vi "Test Data Trimming.vi"() -> ()   [LabVIEW 2018]
panel:
  out "time":dbl
  out "array for saving":sgl[](array[numeric])
  in  "start pixel":i32
  in  "#A-lines per B-line":i32=2048
  in  "#pixels to save":i32=200
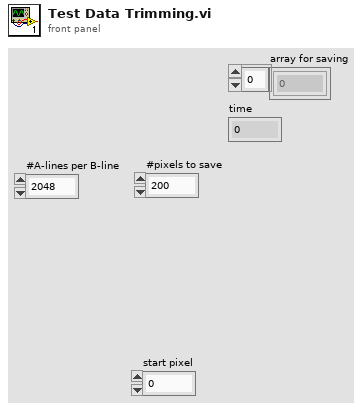
[diagram p1: front panel]
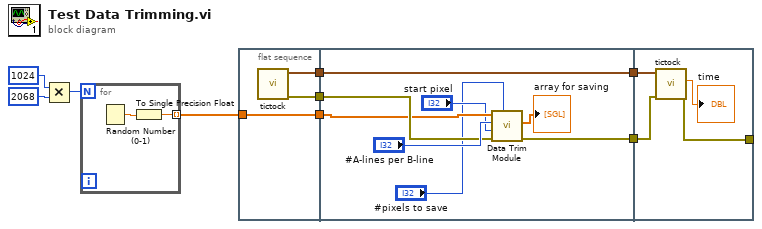
[diagram p0: block diagram]
diagram:
  n1 = Multiply(x=1024, y=2068) -> (x*y=w7:i32)
  n2 = for {
    N: w7 -> [_]
    tunnel: [w10] -> w1 mode=indexing
    n3 = Random Number (0-1)() -> (number: 0 to 1=w11:dbl)
    n4 = To Single Precision Float(number=w11) -> (single precision float=w10:sgl)
  }
  n5 = flat-sequence {
    tunnel: w1 -> [w14]
    tunnel: [w14] -> w6
    tunnel: [w13] -> w4
    tunnel: [w12] -> w3
    tunnel: w6 -> [w18]
    tunnel: [w21] -> w5
    tunnel: w4 -> [w21]
    tunnel: w3 -> [w20]
    tunnel: [w19] -> w2
    tunnel: w5 -> [w26]
    tunnel: w2 -> [w24]
    tunnel: [w23] -> _
    frame #0 {
      n6 = call "tictock.vi"() -> ("error out"=w12:errorcluster, "seconds since 1Jan1904"=w13:timestamp)  [unwired: 9 in, 1 out]
    }
    frame #1 {
      n7 = call "Data Trim Module.vi"("#pixels to save"="#pixels to save", "error in"=w20, "start pixel"="start pixel", "#A-lines"="#A-lines per B-line", "1D Array in"=w18) -> ("error out"=w19:errorcluster, "array for saving"=→"array for saving":sgl[])  [unwired: 4 in, 1 out]
    }
    frame #2 {
      n8 = call "tictock.vi"("error in (no error)"=w24, "seconds since 1Jan1904 2"=w26) -> ("error out"=w23:errorcluster, "Numeric"=→"time":dbl)  [unwired: 7 in, 1 out]
    }
  }
